vi "Byte Buffer.Buffer Subset.Get.vi"(7 "length (-1: rest)":i64=-1, 8 "error in (no error)":errorcluster, 9 "offset (0)":u64, 10 "allocated string in":string, 11 "Byte Buffer in":refnum<class "Byte Buffer.lvclass">) -> (0 "error out":errorcluster, 1 "new buffer offset":u64, 2 "string out":string, 3 "Byte Buffer out":refnum<class "Byte Buffer.lvclass">)   [LabVIEW 2016, in "VeriStand Data.lvlib" / "Byte Buffer.lvclass"]
uses:
  Byte Buffer.lvclass
  Byte Buffer.lvclass/Byte Buffer.ctl
  Memory Management/Memory Management.Handle Return.vi
  VeriStand Data.lvlib
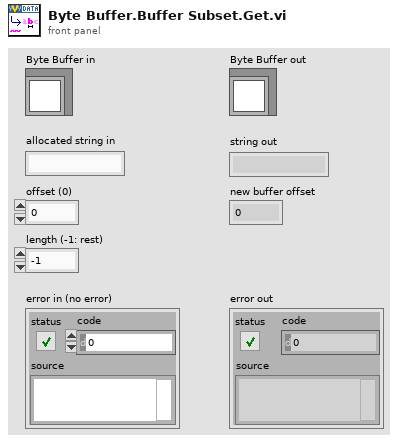
[diagram p1: front panel]
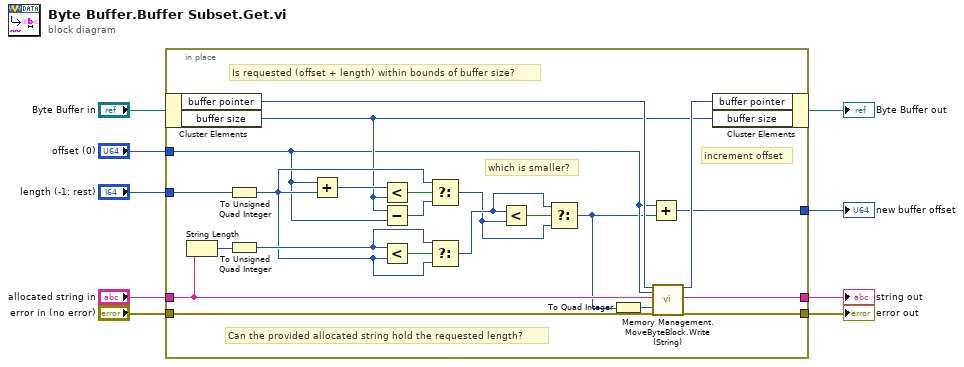
[diagram p0: block diagram]
diagram:
  n1 = in-place {
    in-place-border: "error in (no error)" -> [w31]
    in-place-border: "allocated string in" -> [w28]
    in-place-border: "length (-1: rest)" -> [w25]
    in-place-border: "offset (0)" -> [w11]
    in-place-border: [w24] -> w4
    in-place-border: [w23] -> w3
    in-place-border: [w12] -> w1
    # "increment offset"
    # "which is smaller?"
    # "Can the provided allocated string hold the requested length?"
    # "Is requested (offset + length) within bounds of buffer size?"
    n2 = in-place-cluster #1("Byte Buffer in") -> ("buffer pointer"=w27:u64, "buffer size"=w13:u64)
    n3 = String Length(string=w28) -> (length=w29:i32)
    n4 = To Unsigned Quad Integer(1:w25) -> (0:w16:u64)
    n5 = To Unsigned Quad Integer(1:w29) -> (0:w21:u64)
    n6 = Add(x=w11, y=w16) -> (x+y=w26:u64)
    n7 = Less?(x=w26, y=w13) -> (x < y?=w30:bool)
    n8 = Subtract(x=w13, y=w11) -> (x-y=w15:u64)
    n9 = Less?(x=w21, y=w16) -> (x < y?=w22:bool)
    n10 = Select(t=w16, s=w30, f=w15) -> (s? t:f=w18:u64)
    n11 = Select(t=w21, s=w22, f=w16) -> (s? t:f=w19:u64)
    n12 = Less?(x=w19, y=w18) -> (x < y?=w20:bool)
    n13 = Select(t=w19, s=w20, f=w18) -> (s? t:f=w10:u64)
    n14 = To Quad Integer(1:w10) -> (0:w14:i64)
    n15 = Add(x=w11, y=w10) -> (x+y=w12:u64)
    n16 = call "Memory Management.MoveByteBlock.Write (String).vi"("src ptr in"=w27, "src offset (0)"=w11, "dst in"=w28, "size"=w14, "error in (no error)"=w31) -> ("src ptr out"=w17:u64, "dst out"=w23:string, "error out"=w24:errorcluster)  [unwired: 9 in, 3 out]
    n17 = in-place-cluster #1("buffer pointer"=w17, "buffer size"=w13) -> (→"Byte Buffer out":refnum<class "Byte Buffer.lvclass">)
  }
  "error out" <- w4
  "string out" <- w3
  "new buffer offset" <- w1
